vi "Msg.vi"(7 "Actor in":refnum<class "Actor.lvclass">, 11 "Pop Up Msg in":refnum<class "Pop Up Msg.lvclass">) -> (5 "Actor out":refnum<class "Actor.lvclass">)   [LabVIEW 2021, in "Pop Up.lvlib" / "Pop Up Msg.lvclass"]
uses:
  Pop Up Msg.lvclass
  Actor/Actor/Actor.lvclass
  Pop Up/Pop Up.lvclass
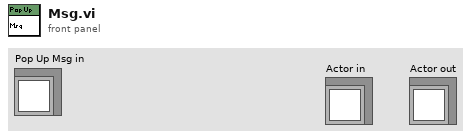
[diagram p1: front panel]
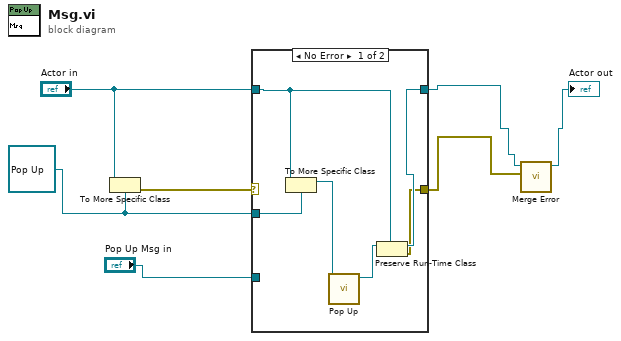
[diagram p0: block diagram]
diagram:
  w5 = refnum<class "Pop Up.lvclass"> refnum ("Pop Up.lvlib:Pop Up.lvclass")
  n1 = To More Specific Class(target class=w5, reference="Actor in") -> (error out=w7:errorcluster)  [unwired: 1 in, 1 out]
  n2 = case shown="No Error" w7 {
    selector: w7 -> [_ w14]
    tunnel: [w9 w15] -> w4
    tunnel: "Actor in" -> [w11 w15]
    tunnel: w5 -> [w13 _]
    tunnel: "Pop Up Msg in" -> [_ _]
    tunnel: [w8 w14] -> w3
    frame No Error {
      n3 = To More Specific Class(target class=w13, reference=w11) -> (specific class reference=w12:refnum<class "Pop Up.lvclass">)  [unwired: 1 in, 1 out]
      n4 = call-dynamic "Pop Up.vi"("Pop Up in"=w12) -> ("Pop Up out"=w10:refnum<class "Pop Up.lvclass">)  [unwired: 10 in]
      n5 = Preserve Run-Time Class(object in=w10, 2:w11) -> (object out=w9:refnum<class "Actor.lvclass">, error out=w8:errorcluster)  [unwired: 1 in]
    }
    frame Error {
    }
  }
  n6 = call-dynamic "Merge Error.vi"("Error"=w3, "Set Error in"=w4) -> ("Set Error out"=→"Actor out":refnum<class "Actor.lvclass">)  [unwired: 9 in]
